vi "Get Metadata.vi"(7 "DLL path":path, 8 "error in (no error)":errorcluster, 11 "session id in":i32) -> (0 "error out":errorcluster, 2 "Metadata":string[][](table), 3 "session id out":i32)   [LabVIEW 2017, in "ONNX Class Library.lvlib"]
doc: "Get Metadata from ONNX"
uses:
  ONNX Class Library.lvlib
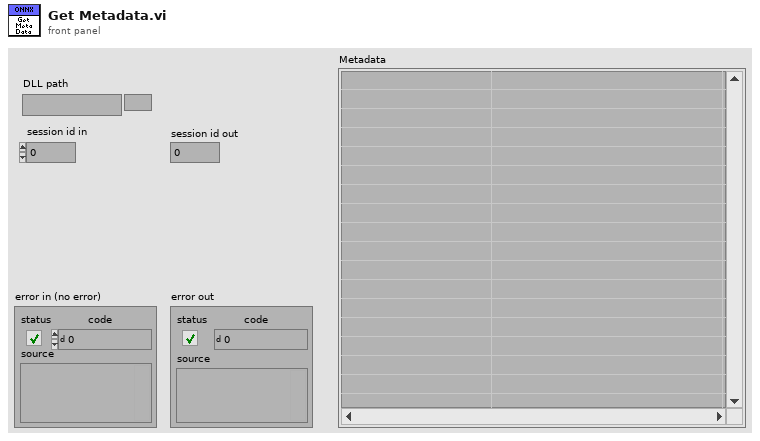
[diagram p1: front panel]
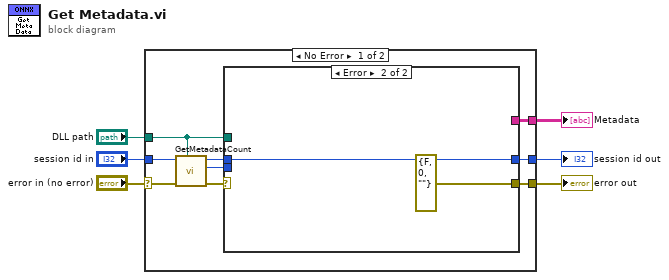
[diagram p0: block diagram]
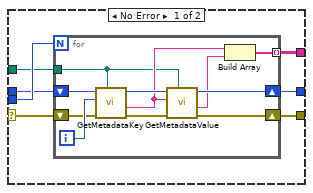
[diagram p2: hidden frame]
diagram:
  n1 = case shown="No Error" "error in (no error)" {
    selector: "error in (no error)" -> [w9 w36]
    tunnel: [w13 _] -> w6
    tunnel: [w12 w36] -> w5
    tunnel: "session id in" -> [w11 w37]
    tunnel: [w10 w37] -> w3
    tunnel: "DLL path" -> [w8 _]
    frame No Error {
      n2 = call "GetMetadataCount.vi"("DLL path"=w8, "error in (no error)"=w9, "session id in"=w11) -> ("error out"=w7:errorcluster, "MetadataCount"=w15:i32, "session id out"=w14:i32)  [unwired: 6 in]
      n3 = case shown="Error" w7 {
        selector: w7 -> [w16 _]
        tunnel: w15 -> [w22 _]
        tunnel: w14 -> [w21 w35]
        tunnel: [w20 _] -> w13
        tunnel: [w19 errorcluster {"status"=FALSE, "code"=0, "source"=""} ("error IO")] -> w12
        tunnel: [w18 w35] -> w10
        tunnel: w8 -> [w17 _]
        frame No Error {
          n4 = for {
            N: w22 -> [_]
            shift-right: [w28] -> w18
            shift-left: w21 -> [w33]
            shift-right: [w27] -> w19
            shift-left: w16 -> [w31]
            tunnel: [w24] -> w20 mode=indexing
            tunnel: w17 -> [w23]
            i -> [w32]
            n5 = call "GetMetadataKey.vi"("DLL path"=w23, "error in (no error)"=w31, "index"=w32, "session id in"=w33) -> ("error out"=w29:errorcluster, "MetadataKey"=w26:string, "session id out"=w30:i32)  [unwired: 5 in]
            n6 = call "GetMetadataValue.vi"("DLL path"=w23, "error in (no error)"=w29, "key"=w26, "session id in"=w30) -> ("error out"=w27:errorcluster, "MetadataValue"=w25:string, "session id out"=w28:i32)  [unwired: 5 in]
            n7 = Build Array(w26, w25) -> (w24:string[])
          }
        }
        frame Error {
        }
      }
    }
    frame Error {
    }
  }
  "Metadata" <- w6
  "error out" <- w5
  "session id out" <- w3
